vi "Initialize.vi"(7 "Comm Interface":T2, 8 "error in (no error)":errorcluster {"code" format="%x"}, 9 "ethernetSetting":T1, 10 "timeout":u32, 11 "deviceId":i32) -> (0 "error out":errorcluster {"code" format="%x"})   [LabVIEW 2020, in "Keyence CL-3000.lvlib"]
doc: "This function establishes a connection with the controller so that the library can communicate with a USB-connected or Ethernet-connected controller."
uses:
  Keyence CL-3000.lvlib
  enums/Comm Interface.ctl
  clusters/CL3IF_ETHERNET_SETTING.ctl
  Private/enums/Function Name.ctl
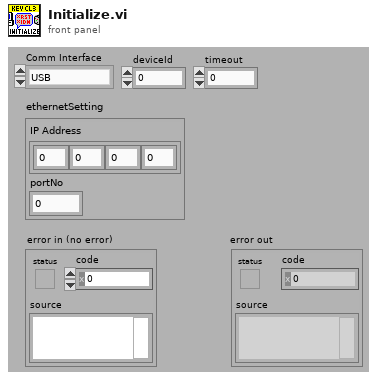
[diagram p1: front panel]
types:
  T1 = typedef "Keyence CL-3000.lvlib/CL3IF_ETHERNET_SETTING.ctl" = cluster{"IP Address":cluster{"IP1":u8, "IP2":u8, "IP3":u8, "IP4":u8}, "portNo":u32}
  T2 = typedef "Keyence CL-3000.lvlib/Comm Interface.ctl" = enum8{"USB", "ETHERNET"}
  T3 = typedef "Keyence CL-3000.lvlib/Function Name.ctl" = enum16{"Initialize", "Close", "CL3IF_GetMeasurementData", "CL3IF_GetTrendIndex", "CL3IF_GetTrendData", "CL3IF_GetStorageIndex", "CL3IF_GetStorageData", "CL3IF_AutoZeroMulti", "CL3IF_AutoZeroGroup", "CL3IF_TimingMulti", "CL3IF_TimingGroup", "CL3IF_ResetMulti", "CL3IF_ResetGroup", "CL3IF_LightControl", "CL3IF_MeasurementControl", "CL3IF_SwitchProgram", "CL3IF_GetProgramNo", "CL3IF_StartStorage", "CL3IF_StopStorage", "CL3IF_ClearStorageData", "CL3IF_GetPulseCount", "CL3IF_ResetPulseCount", "CL3IF_GetLightWaveform"}
  T4 = cluster{"ethernetSetting":T1, "reserved[2]":cluster{u8, u8}}
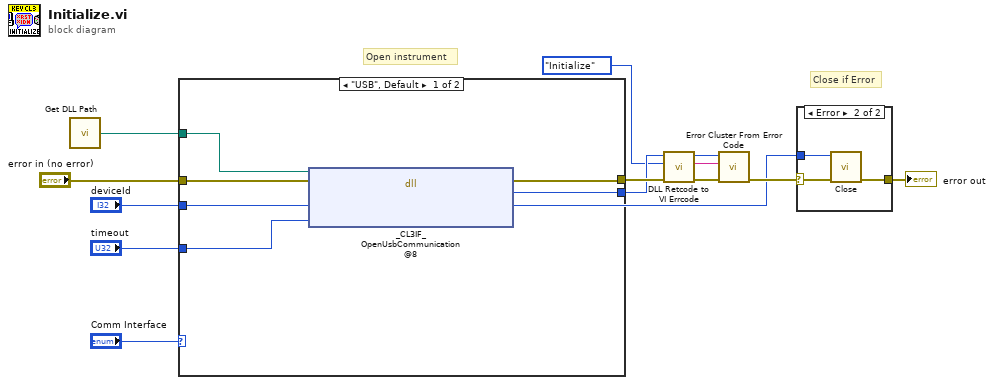
[diagram p0: block diagram]
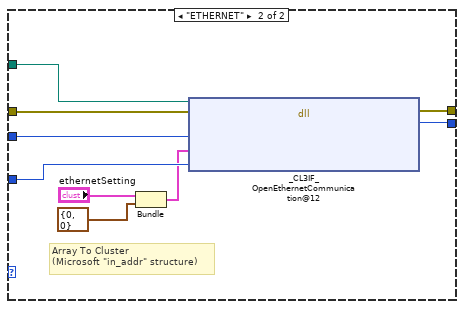
[diagram p2: hidden frame]
diagram:
  # "Close if Error"
  # "Open instrument"
  n1 = call "Get DLL Path.vi"() -> ("DLL Path"=w5:path)  [unwired: 1 in]
  n2 = case shown="\"USB\", Default" "Comm Interface" {
    tunnel: "error in (no error)" -> [w19 w28]
    tunnel: [w18 w27] -> w10
    tunnel: [w17 w26] -> w9
    tunnel: w5 -> [w16 w25]
    tunnel: "deviceId" -> [w15 w24]
    tunnel: "timeout" -> [w14 w23]
    frame "USB", Default {
      n3 = dll-call lib="C:/Program Files (x86)/National Instruments/LabVIEW 2018/instr.lib/Keyence CL-3000/CL3_IF.dll" fn="_CL3IF_OpenUsbCommunication@8"(path in=w16, error in=w19, "deviceId"=w15, "timeout"=w14) -> (error out=w18:errorcluster, "RC"=w17:i32)  [unwired: 3 in, 1 out]
    }
    frame "ETHERNET" {
      # "Array To Cluster\n(Microsoft \"in_addr\" structure)"
      n4 = Bundle("ethernetSetting"="ethernetSetting", "reserved[2]"=cluster{u8, u8} {0, 0}) -> (w20:T4)  [unwired: 1 in]
      n5 = dll-call lib="C:/Program Files (x86)/National Instruments/LabVIEW 2018/instr.lib/Keyence CL-3000/CL3_IF.dll" fn="_CL3IF_OpenEthernetCommunication@12"(path in=w25, error in=w28, "deviceId"=w24, "OpenParam"=w20, "timeout"=w23) -> (error out=w27:errorcluster, "RC"=w26:i32)  [unwired: 4 in, 1 out]
    }
  }
  n6 = call "DLL Retcode to VI Errcode.vi"("error in (no error)"=w10, "Function Name"=Function_Name."Initialize", "DLL Retcode"=w9) -> ("error out"=w8:errorcluster, "ErrorMessage"=w2:string, "VI Errcode"=w7:i32)  [unwired: 6 in]
  n7 = call <vilib>:"Error Cluster From Error Code.vi"("error in (no error)"=w8, "error message (\"\")"=w2, "error code (0)"=w7) -> ("error out"=w6:errorcluster)  [unwired: 6 in]
  n8 = case shown="Error" w6 {
    selector: w6 -> [w29 w31]
    tunnel: [w29 w32] -> w13
    tunnel: "deviceId" -> [_ w30]
    frame No Error {
    }
    frame Error {
      n9 = call "Close.vi"("error in (no error)"=w31, "deviceId"=w30) -> ("error out"=w32:errorcluster)  [unwired: 9 in]
    }
  }
  "error out" <- w13
